vi "save file data.vi"(8 "error in":errorcluster, 10 "format":T1, 11 "Path":path) -> (0 "error out":errorcluster)   [LabVIEW 2025, in "CEF.lvlib"]
doc: "Saves a file containing the <b>base file format.ctl</b>, which is a tuple of version and data.Copyright 2017 National Instruments Corporation\n\nLicensed under the Apache License, Version 2.0 (the \"License\"); you may not use this file except in compliance with the License. You may obtain a copy of the License at http://www.apache.org/licenses/LICENSE-2.0\nUnless required by applicable law or agreed to in writing, software distributed under the License is distributed on an \"AS IS\" BASIS, WITHOUT WARRANTIES OR CONDITIONS OF ANY KIND, either express or implied. See the License for the specific language governing permissions and limitations under the License."
uses:
  CEF.lvlib
  base file format.ctl
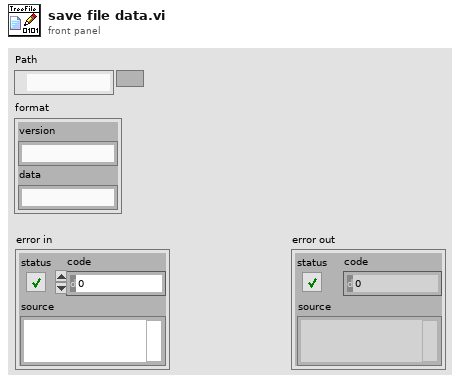
[diagram p1: front panel]
types:
  T1 = typedef "CEF.lvlib/base file format.ctl" = cluster{"version":string, "data":string}
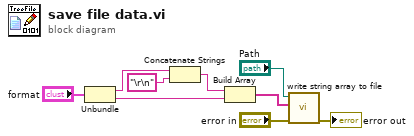
[diagram p0: block diagram]
diagram:
  n1 = Unbundle("format") -> ("version"=w8:string, "data"=w1:string)
  n2 = Concatenate Strings(w8, "\r\n" ("String")) -> (w6:string)
  n3 = Build Array(w6, w1) -> (w2:string[])
  n4 = call "write string array to file.vi"("error in"="error in", "strings"=w2, "file path"="Path") -> ("error out"=→"error out":errorcluster)  [unwired: 8 in]
